vi "Switch Build Key Array for Config.vi"(8 "error in (no error)":errorcluster, 9 "Switch Test Parameters":T2, 10 "Key Array In":T6, 11 "Connection Refnum":T1) -> (0 "error out":errorcluster, 1 "$$INITCODE$$":string, 2 "Key Array Out":T6, 3 "Connection Refnum":T1)   [LabVIEW 2011]
uses:
  ITK EXT/utils/keyedarr.llb/Keyed Array.ctl
  TypeDefs/Switch Test Parameters.ctl
  TypeDefs/Switch Stimulus Parameters.ctl
  TypeDefs/Switch Type.ctl
  TypeDefs/Switch Instrument Info.ctl
  Summitek EXT/ODBC/SQL Controls/Connection Refnum.ctl
  ITK EXT/utils/strutil.llb/Case Matching.ctl
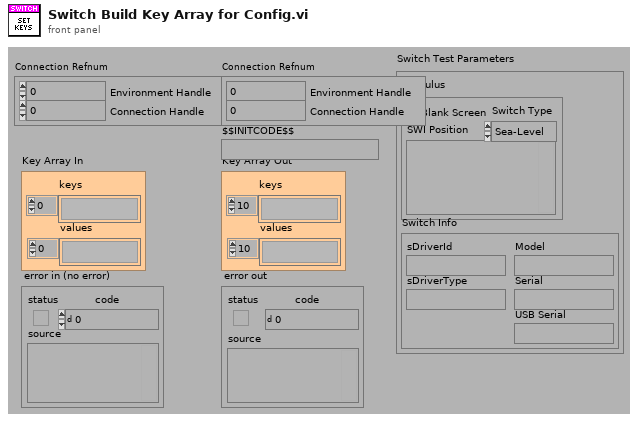
[diagram p1: front panel]
types:
  T1 = typedef "Connection Refnum.ctl" = cluster{"Environment Handle":i32, "Connection Handle":i32}
  T2 = typedef "Switch Test Parameters.ctl" = cluster{"Stimulus":T3, "Switch Info":T5}
  T3 = typedef "Switch Stimulus Parameters.ctl" = cluster{"Blank Screen":bool, "SWI Position":variant, "Switch Type":T4}
  T4 = typedef "Switch Type.ctl" = enum16{"Sea-Level", "Simulator", "SI-0206-SW", "SI-0309-SW", "SI-0310-SW", "Front End"}
  T5 = typedef "Switch Instrument Info.ctl" = cluster{"sDriverId":string, "sDriverType":string, "Model":string, "Serial":string, "USB Serial":string}
  T6 = typedef "Keyed Array.ctl" = cluster{"keys":string[], "values":string[]}
  T7 = typedef "Case Matching.ctl" = enum16{"a != A", "a == A", "system"}
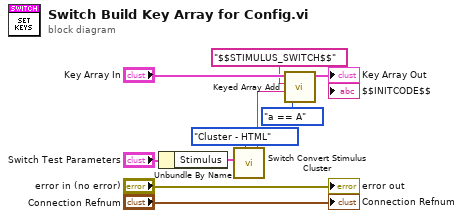
[diagram p0: block diagram]
diagram:
  n1 = Unbundle By Name("Switch Test Parameters") -> ("Stimulus"=w8:T3)
  n2 = call "Switch Convert Stimulus Cluster.vi"("Conversion"=enum16{"Cluster - HTML", "HTML - Cluster"}."Cluster - HTML", "Stimulus Cluster In"=w8) -> ("Stumulus HTML Out"=w3:string)  [unwired: 5 in, 1 out]
  n3 = call "Keyed Array Add.vi"("case matching (sensitive)"=Case_Matching."a == A", "value"=w3, "key"="$$STIMULUS_SWITCH$$", "array in"="Key Array In") -> ("array out"=→"Key Array Out":T6)  [unwired: 3 out]
  "error out" <- "error in (no error)"
  "Connection Refnum" <- "Connection Refnum"
